vi "Read Choices.vi"(8 "error in (no error)":errorcluster, 11 "NT Enum in":refnum<class "NT Enum.lvclass">) -> (0 "error out":errorcluster, 2 "choices":string[](array[string]), 3 "NT Enum out":refnum<class "NT Enum.lvclass">)   [LabVIEW 2020, in "PV Access.lvlib" / "PV Data.lvlib" / "NT Enum.lvclass"]
uses:
  NT Enum.lvclass
  NT Enum.lvclass/NT Enum.ctl
  8f5eaf6c-17e8-446a-a8c9-9407631de8a9.vi
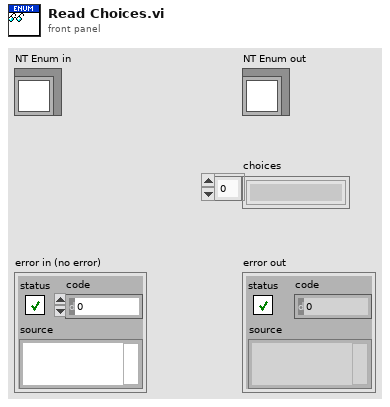
[diagram p1: front panel]
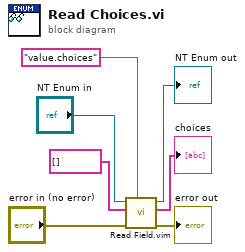
[diagram p0: block diagram]
diagram:
  n1 = call "Read Field.vim"("field"="value.choices", "error in"="error in (no error)", "default value"=string[] [], "Base Interface in"="NT Enum in") -> ("error out"=→"error out":errorcluster, "value"=→"choices":string[], "Base Interface out"=→"NT Enum out":refnum<class "NT Enum.lvclass">)  [unwired: 5 in]
